vi "Eurotherm - Read I Term.vi"(0 "Eurotherm Setup In":T1={"Communication"={"Com Port"=1, "Address"=1, "Baud Rate"=9600}, "Name"="", "Enable"=FALSE, "Max Set Point"=0.0, "Min Set Point"=0.0, "Units"="", "Graph Data"=0, "Sensor type"=enum."RhFe", "Calibration File Path"=path "", "Conversion Type"=enum."Linear"} {"Min Set Point" format="%.3f"; "Max Set Point" format="%.3f"; "Communication"."Baud Rate" items=["300"=300, "600"=600, "1200"=1200, "2400"=2400, "4800"=4800, "9600 (default)"=9600, "19200"=19200, "38400"=38400, "57600"=57600, "76800"=76800, "115200"=115200, "230400"=230400]; "Communication"."Com Port" min=1 max=255; "Communication"."Address" min=1 max=99}, 11 "error in (no error)":errorcluster) -> (4 "Eurotherm Setup Out":T1={"Communication"={"Com Port"=1, "Address"=1, "Baud Rate"=9600}, "Name"="", "Enable"=FALSE, "Max Set Point"=0.0, "Min Set Point"=0.0, "Units"="", "Graph Data"=0, "Sensor type"=enum."RhFe", "Calibration File Path"=path "", "Conversion Type"=enum."Linear"} {"Min Set Point" format="%.3f"; "Max Set Point" format="%.3f"; "Communication"."Baud Rate" items=["300"=300, "600"=600, "1200"=1200, "2400"=2400, "4800"=4800, "9600 (default)"=9600, "19200"=19200, "38400"=38400, "57600"=57600, "76800"=76800, "115200"=115200, "230400"=230400]; "Communication"."Com Port" min=1 max=255; "Communication"."Address" min=1 max=99}, 8 "I":dbl, 15 "error out":errorcluster)   [LabVIEW 2011]
uses:
  Eurotherm - Controls/Eurotherm - Setup.ctl
  Eurotherm - Controls/Eurotherm - Communication.ctl
  Common/Utilities/Controls - Com Ports/Com Port - Numeric.ctl
  Eurotherm - Controls/Eurotherm - Address.ctl
  Common/Utilities/Controls - Com Ports/Com Port - Baud Rate.ctl
  Common/Utilities - System/Sensors/Sensors - Controls/Sensors - Temperature Sensor Type.ctl
  Common/Utilities - System/Sensors/Sensors - Controls/Sensors - Conversion Type.ctl
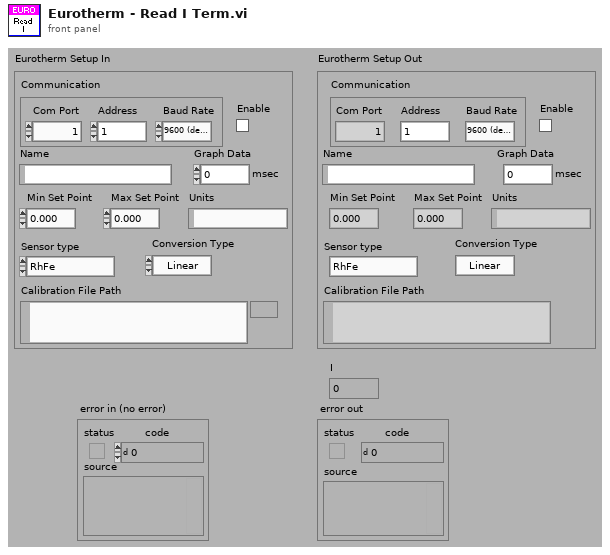
[diagram p1: front panel]
types:
  T1 = typedef "Eurotherm - Setup.ctl" = cluster{"Communication":T2, "Name":string, "Enable":bool, "Max Set Point":dbl, "Min Set Point":dbl, "Units":string, "Graph Data":u32, "Sensor type":T6, "Calibration File Path":path, "Conversion Type":T7}
  T2 = typedef "Eurotherm - Communication.ctl" = cluster{"Com Port":T3, "Address":T4, "Baud Rate":T5}
  T3 = typedef "Com Port - Numeric.ctl" = i32
  T4 = typedef "Eurotherm - Address.ctl" = u8
  T5 = typedef "Com Port - Baud Rate.ctl" = u32
  T6 = typedef "Sensors - Temperature Sensor Type.ctl" = enum16{"RhFe", "Pt", "K type thermocouple", "W5 type thermocouple", "No Conversion"}
  T7 = typedef "Sensors - Conversion Type.ctl" = enum16{"Linear", "Spline"}
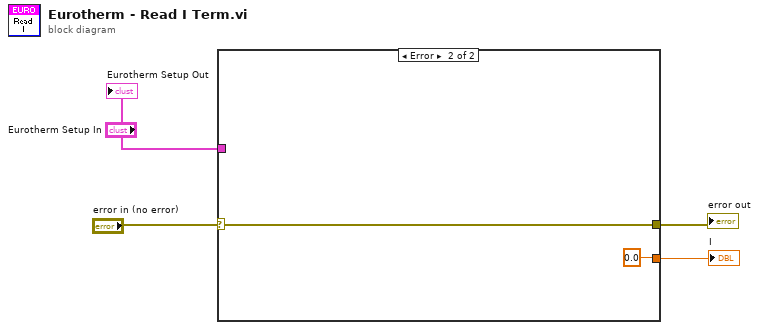
[diagram p0: block diagram]
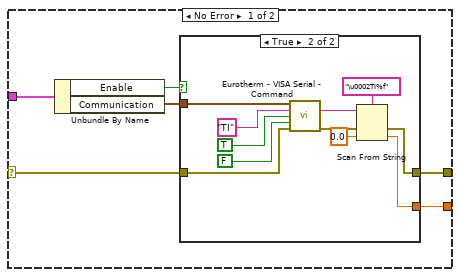
[diagram p2: hidden frame]
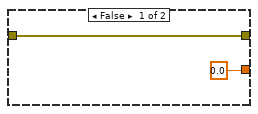
[diagram p3: hidden frame]
diagram:
  n1 = case shown="Error" "error in (no error)" {
    selector: "error in (no error)" -> [w10 w25]
    tunnel: [w9 w25] -> w3
    tunnel: [w6 0.0 ("default value 1")] -> w2
    tunnel: "Eurotherm Setup In" -> [w5 _]
    frame No Error {
      n2 = Unbundle By Name(w5) -> ("Enable"=w7:bool, "Communication"=w8:T2)
      n3 = case shown="True" w7 {
        tunnel: w10 -> [w12 w23]
        tunnel: [w12 w16] -> w9
        tunnel: w8 -> [_ w19]
        tunnel: [0.0 ("default value 1") w13] -> w6
        frame False {
        }
        frame True {
          n4 = call "Eurotherm - VISA Serial - Command.vi"("VISA resource name In (String)"=w19, "Command"="TI", "Read Reply"=TRUE, "Close Session"=FALSE, "error in (no error)"=w23) -> ("Reply"=w15:string, "error out"=w17:errorcluster)  [unwired: 8 in, 1 out]
          n5 = Scan From String(format string="\u0002TI%f", input string=w15, error in=w17, default 1=0.0 ("default value 1")) -> (error out=w16:errorcluster, output 1=w13:dbl)  [unwired: 1 in, 2 out]
        }
      }
    }
    frame Error {
    }
  }
  "error out" <- w3
  "I" <- w2
  "Eurotherm Setup Out" <- "Eurotherm Setup In"
